vi "RAW Event.vi"(0 "Connection Info":T1, 5 "State Variables":T3, 7 "Address Lookup Table":variant, 9 "Identifier":u32 format="%08x", 11 "Data":u8[](array[numeric])=[0, 0, 0, 0, 0, 0, 0, 0], 12 "Error Q":refnum<queue>, 13 "VI Ref":refnum<vi>) -> (4 "Connection Info Out":T1, 8 "Address Lookup Table Out":variant)   [LabVIEW 2015, in "J1939 Addon Shared.lvlib"]
uses:
  J1939 Addon Shared.lvlib
  Types/Private Data.ctl
  Types/Error Cluster.ctl
  Types/Error Types.ctl
  STM/TCP/stm_TCP Connection Info.ctl
  STM/_SubVIs/stm_MetaDataElement.ctl
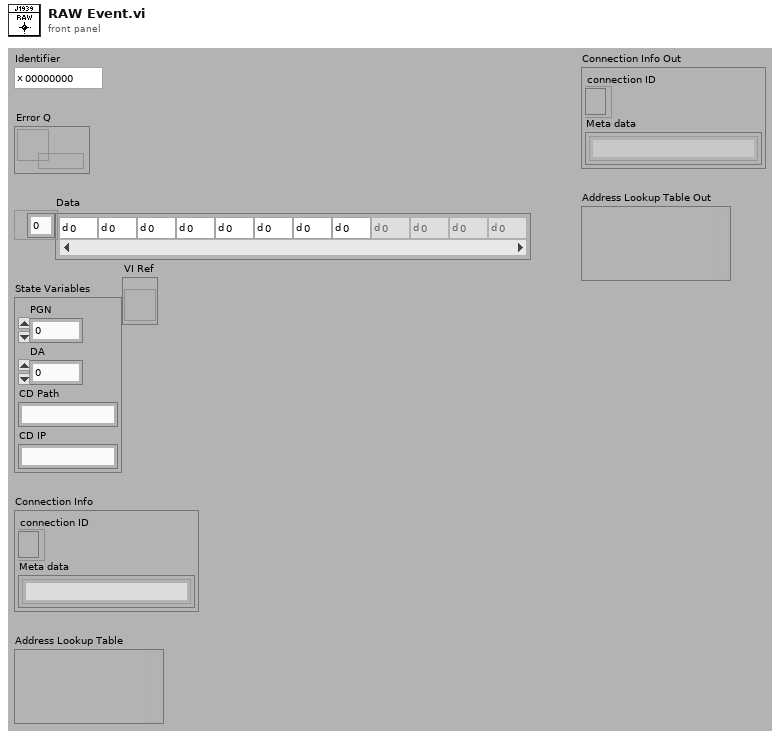
[diagram p1: front panel]
types:
  T1 = typedef "J1939 Addon Shared.lvlib/stm_TCP Connection Info.ctl" = cluster{"connection ID":refnum<k5>, "Meta data":T2[]}
  T2 = typedef "J1939 Addon Shared.lvlib/stm_MetaDataElement.ctl" = string
  T3 = typedef "J1939 Addon Shared.lvlib/Private Data.ctl" = cluster{"PGN":u32, "DA":u8, "CD Path":string, "CD IP":string}
  T4 = typedef "J1939 Addon Shared.lvlib/Error Types.ctl" = enum16{"Request", "RAW Generation", "Clear Active DTCs", "Clear Previous DTCs", "Addresses", "TLAs", "Get Active DTCs", "Get Previous DTCs"}
  T5 = typedef "J1939 Addon Shared.lvlib/Error Cluster.ctl" = cluster{"error out":errorcluster, "Enum":T4, "Address":u8, "Timestamp":timestamp}
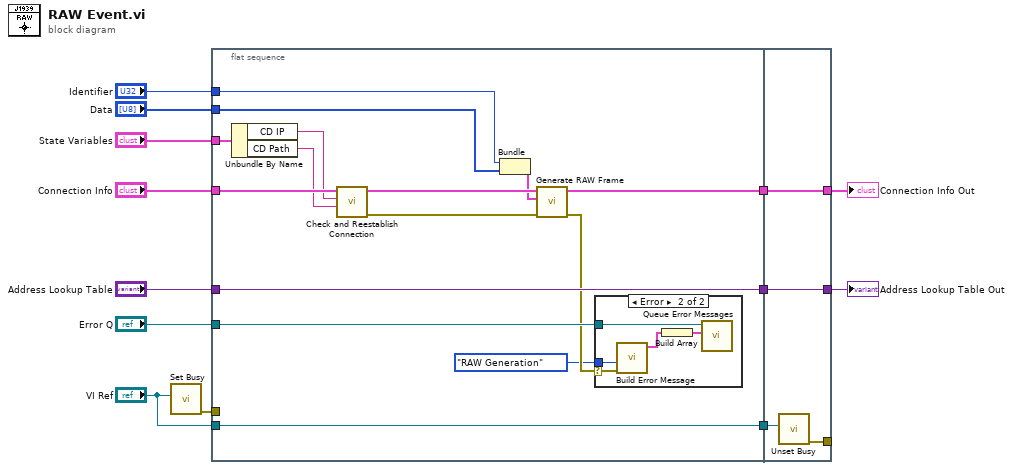
[diagram p0: block diagram]
diagram:
  n1 = call <vilib>:"Set Busy.vi"("VI reference (current VI)"="VI Ref") -> ("error out"=w7:errorcluster)  [unwired: 9 in, 1 out]
  n2 = flat-sequence {
    tunnel: "Connection Info" -> [w28]
    tunnel: w7 -> [_]
    tunnel: [w16] -> w13
    tunnel: [w24] -> w12
    tunnel: "Address Lookup Table" -> [w24]
    tunnel: "Error Q" -> [w23]
    tunnel: "State Variables" -> [w20]
    tunnel: "VI Ref" -> [w17]
    tunnel: [w17] -> w3
    tunnel: "Identifier" -> [w15]
    tunnel: "Data" -> [w14]
    tunnel: [w37] -> w6
    tunnel: w13 -> [w37]
    tunnel: [w36] -> _
    tunnel: [w35] -> w8
    tunnel: w12 -> [w35]
    tunnel: w3 -> [w34]
    frame #0 {
      n3 = Unbundle By Name(w20) -> ("CD IP"=w19:string, "CD Path"=w18:string)
      n4 = call "Check and Reestablish Connection.vi"("CD Path"=w18, "IP Address"=w19, "Connection Info"=w28) -> ("error out"=w27:errorcluster, "Connection Info Out"=w26:T1)  [unwired: 7 in]
      n5 = Bundle("Identifier"=w15, "Data"=w14) -> (w25:cluster{"Identifier":u32, "Data":u8[]})  [unwired: 1 in]
      n6 = call "Generate RAW Frame.vi"("error in (no error)"=w27, "Data to Send"=w25, "Connection Info"=w26) -> ("error out"=w22:errorcluster, "Connection Info Out"=w16:T1)  [unwired: 7 in]
      n7 = case shown="Error" w22 {
        selector: w22 -> [_ w32]
        tunnel: w23 -> [_ w33]
        tunnel: Error_Types."RAW Generation" ("Enum") -> [_ w29]
        frame No Error {
        }
        frame Error {
          n8 = call "Build Error Message.vi"("error IO"=w32, "Enum"=w29) -> ("Error Cluster"=w31:T5)  [unwired: 9 in]
          n9 = Build Array(w31) -> (w30:T5[])
          n10 = call "Queue Error Messages.vi"("Error Array"=w30, "queue out"=w33) -> ()  [unwired: 9 in, 1 out]
        }
      }
    }
    frame #1 {
      n11 = call <vilib>:"Unset Busy.vi"("VI reference (current VI)"=w34) -> ("error out"=w36:errorcluster)  [unwired: 10 in]
    }
  }
  "Address Lookup Table Out" <- w8
  "Connection Info Out" <- w6
